vi "HumanExecDriveMode.vi"(4 "Enable Field Oriented Drive":bool, 5 "AutoSpeakerAngle":dbl, 6 "State":i32, 7 "Rotation":dbl, 8 "Right X":dbl, 9 "Right Y":dbl, 10 "Left X":dbl, 11 "Left Y":dbl) -> (1 "AMotorDemand":dbl, 2 "YMotorDemand":dbl, 3 "XMotorDemand":dbl)   [LabVIEW 2023]
uses:
  HumanGlobal.vi
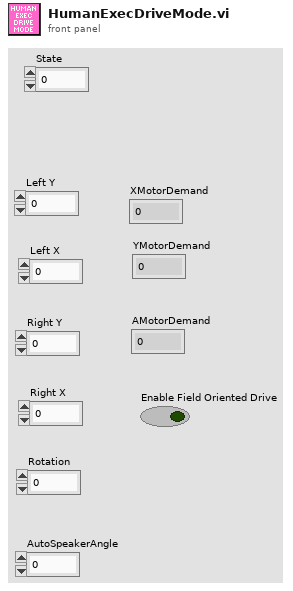
[diagram p1: front panel]
types:
  T1 = enum16{"SpeakerLeft", "SpeakerCenter", "SpeakerRight", "Amp", "Source", "StageLeft", "StageCenter", "StageRight"}
  T2 = typedef "HumanDriveModeENUM.ctl" = enum16{"0 - Normal Swerve", "1 - Auto traj  - Left Speaker", "2 - Auto traj - Center Speaker", "3 - Auto traj - Speaker Right", "4 - Auto traj - Amp", "5 - Auto traj - Source", "6 - Auto traj -  Left Stage", "7 - Auto traj - Center Stage", "8 - Auto traj - Right Stage"}
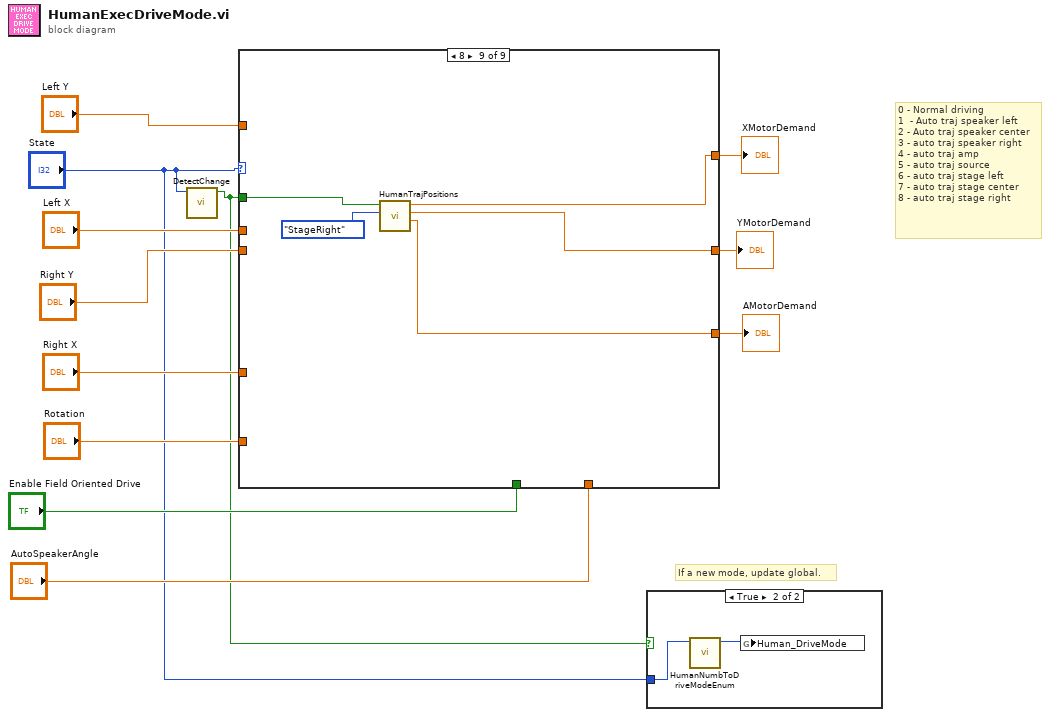
[diagram p0: block diagram]
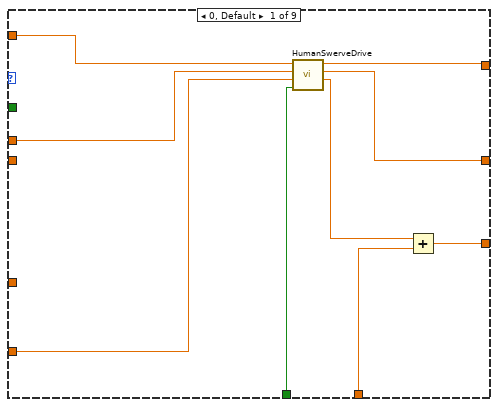
[diagram p3: hidden frame]
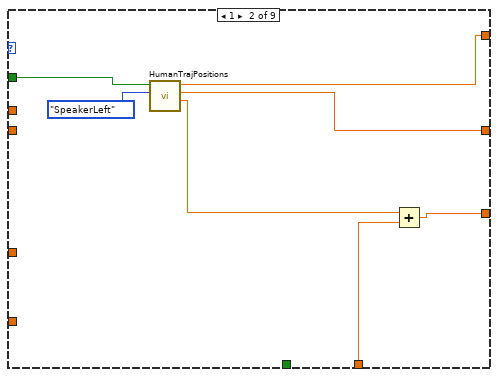
[diagram p4: hidden frame]
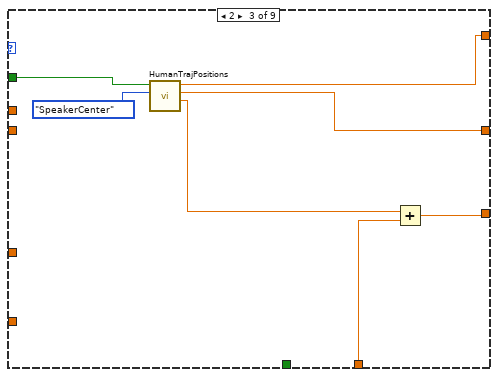
[diagram p5: hidden frame]
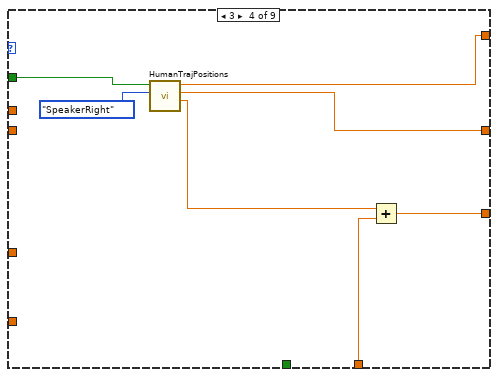
[diagram p6: hidden frame]
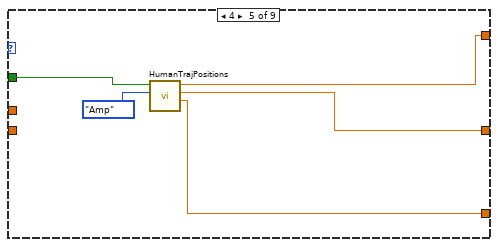
[diagram p7: hidden frame]
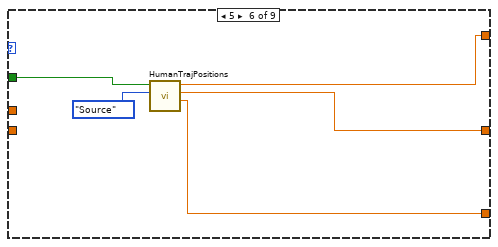
[diagram p8: hidden frame]
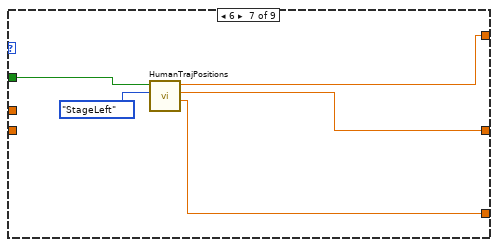
[diagram p9: hidden frame]
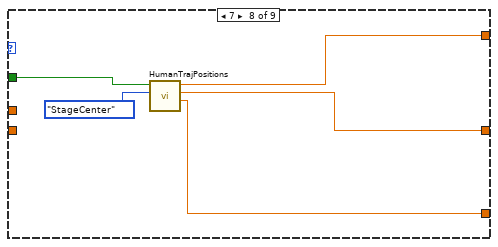
[diagram p10: hidden frame]
diagram:
  # "If a new mode, update global."
  # "0 - Normal driving\n1  - Auto traj speaker left \n2 - Auto traj speaker center\n3 - auto traj speaker right \n4 - auto traj amp\n5 - auto traj source\n6 - auto traj stage left\n7 - auto traj stage center\n8 - auto traj stage right"
  n1 = call "DetectChange.vi"("Value"="State") -> ("Changed"=w2:bool)  [unwired: 10 in]
  n2 = case shown="8" "State" {
    tunnel: "Left Y" -> [w21 _ _ _ _ _ _ _ _]
    tunnel: "Right X" -> [_ _ _ _ _ _ _ _ _]
    tunnel: [w18 w27 w34 w41 w46 w51 w56 w61 w66] -> w10
    tunnel: [w17 w26 w33 w40 w45 w50 w55 w60 w65] -> w9
    tunnel: "Right Y" -> [_ _ _ _ _ _ _ _ _]
    tunnel: w2 -> [_ w28 w35 w42 w47 w52 w57 w62 w67]
    tunnel: "Left X" -> [w20 _ _ _ _ _ _ _ _]
    tunnel: "Rotation" -> [w19 _ _ _ _ _ _ _ _]
    tunnel: [w13 w23 w30 w37 w44 w49 w54 w59 w64] -> w5
    tunnel: "Enable Field Oriented Drive" -> [w16 _ _ _ _ _ _ _ _]
    tunnel: "AutoSpeakerAngle" -> [w15 w22 w31 w36 _ _ _ _ _]
    frame 0, Default {
      n3 = call "HumanSwerveDrive.vi"("Enable Field Oriented Drive"=w16, "Rotation"=w19, "Y"=w20, "X"=w21) -> ("A"=w14:dbl, "Y"=w17:dbl, "X"=w18:dbl)  [unwired: 5 in]
      n4 = Add(x=w14, y=w15) -> (x+y=w13:dbl)
    }
    frame 1 {
      n5 = call "HumanTrajPositions.vi"("FieldPos"=T1."SpeakerLeft", "Init"=w28) -> ("vAngular"=w24:dbl, "vY"=w26:dbl, "vX"=w27:dbl)  [unwired: 7 in]
      n6 = Add(x=w24, y=w22) -> (x+y=w23:dbl)
    }
    frame 2 {
      n7 = call "HumanTrajPositions.vi"("FieldPos"=T1."SpeakerCenter", "Init"=w35) -> ("vAngular"=w29:dbl, "vY"=w33:dbl, "vX"=w34:dbl)  [unwired: 7 in]
      n8 = Add(x=w29, y=w31) -> (x+y=w30:dbl)
    }
    frame 3 {
      n9 = call "HumanTrajPositions.vi"("FieldPos"=T1."SpeakerRight", "Init"=w42) -> ("vAngular"=w38:dbl, "vY"=w40:dbl, "vX"=w41:dbl)  [unwired: 7 in]
      n10 = Add(x=w38, y=w36) -> (x+y=w37:dbl)
    }
    frame 4 {
      n11 = call "HumanTrajPositions.vi"("FieldPos"=T1."Amp", "Init"=w47) -> ("vAngular"=w44:dbl, "vY"=w45:dbl, "vX"=w46:dbl)  [unwired: 7 in]
    }
    frame 5 {
      n12 = call "HumanTrajPositions.vi"("FieldPos"=T1."Source", "Init"=w52) -> ("vAngular"=w49:dbl, "vY"=w50:dbl, "vX"=w51:dbl)  [unwired: 7 in]
    }
    frame 6 {
      n13 = call "HumanTrajPositions.vi"("FieldPos"=T1."StageLeft", "Init"=w57) -> ("vAngular"=w54:dbl, "vY"=w55:dbl, "vX"=w56:dbl)  [unwired: 7 in]
    }
    frame 7 {
      n14 = call "HumanTrajPositions.vi"("FieldPos"=T1."StageCenter", "Init"=w62) -> ("vAngular"=w59:dbl, "vY"=w60:dbl, "vX"=w61:dbl)  [unwired: 7 in]
    }
    frame 8 {
      n15 = call "HumanTrajPositions.vi"("FieldPos"=T1."StageRight", "Init"=w67) -> ("vAngular"=w64:dbl, "vY"=w65:dbl, "vX"=w66:dbl)  [unwired: 7 in]
    }
  }
  "XMotorDemand" <- w10
  "YMotorDemand" <- w9
  "AMotorDemand" <- w5
  n16 = case shown="True" w2 {
    tunnel: "State" -> [_ w69]
    frame False {
    }
    frame True {
      n17 = call "HumanNumbToDriveModeEnum.vi"("DriveModeValue"=w69) -> ("DriveMode"=w68:T2)  [unwired: 10 in]
      n18 = global write "HumanGlobal.vi" "Human_DriveMode"(w68) -> ()
    }
  }
